vi "Read timestamp.vi"(8 "error in (no error)":errorcluster, 11 "AnalysisListItems in":refnum<class "AnalysisListItems.lvclass">) -> (0 "error out":errorcluster, 2 "timestamp":timestamp, 3 "AnalysisListItems out":refnum<class "AnalysisListItems.lvclass">)   [LabVIEW 2018, in "AnalysisListItems.lvclass"]
uses:
  AnalysisListItems.lvclass
  AnalysisListItems.lvclass/AnalysisListItems.ctl
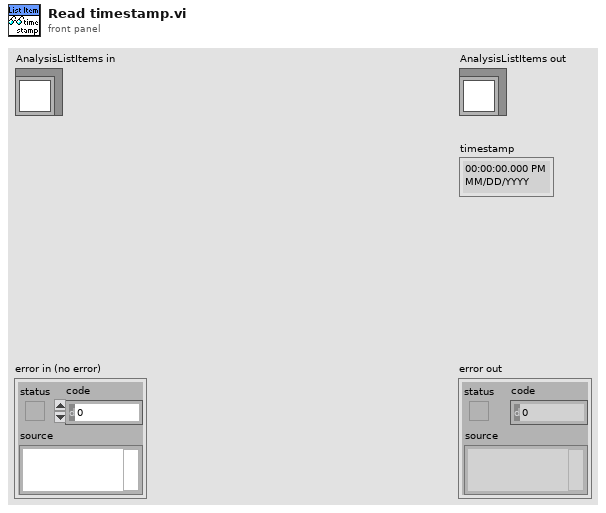
[diagram p1: front panel]
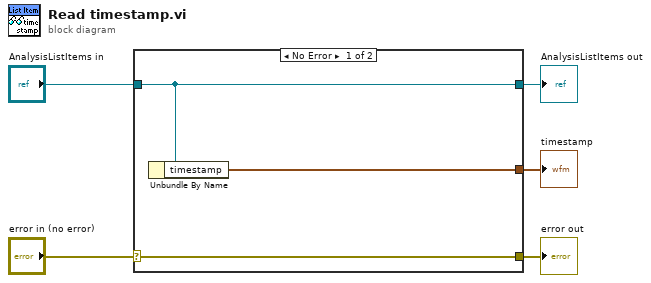
[diagram p0: block diagram]
diagram:
  n1 = case shown="No Error" "error in (no error)" {
    selector: "error in (no error)" -> [w8 w9]
    tunnel: [w8 w9] -> w4
    tunnel: [w7 w10] -> w2
    tunnel: "AnalysisListItems in" -> [w7 w10]
    tunnel: [w6 _] -> w1
    frame No Error {
      n2 = Unbundle By Name(w7) -> ("timestamp"=w6:timestamp)
    }
    frame Error {
    }
  }
  "error out" <- w4
  "AnalysisListItems out" <- w2
  "timestamp" <- w1
